vi "Get Product Info.vi"(8 "error in (no error)":errorcluster, 11 "Name":string) -> (0 "error out":errorcluster, 2 "success?":bool, 3 "Product Info":T1)   [LabVIEW 2020, in "SQLITE Inventory.lvlib"]
doc: "Gets the information of a single product query."
uses:
  SQLITE Inventory.lvlib
  Invetory Data Type.ctl
  <vilib>/drjdpowell/SQLite Library/SQL Connection/Open (path).vi
  <vilib>/drjdpowell/SQLite Library/SQL Connection/Open (string).vi
  <vilib>/AdvancedString/Path To Command Line String.vi
  <vilib>/drjdpowell/SQLite Library/SQL Connection/Execute SQL (Single Integer).vi
  <vilib>/drjdpowell/SQLite Library/SQL Connection/Connection.lvclass
  <vilib>/drjdpowell/SQLite Library/SQLite.lvlib
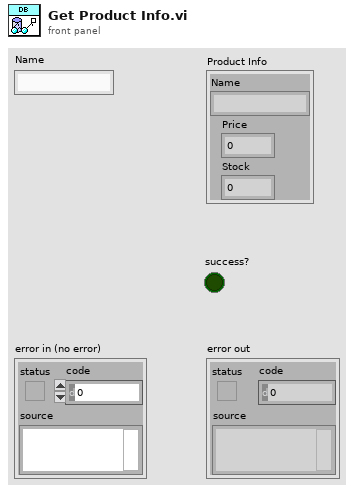
[diagram p1: front panel]
types:
  T1 = typedef "Invetory Data Type.ctl" = cluster{"Name":string, "Price":dbl, "Stock":dbl}
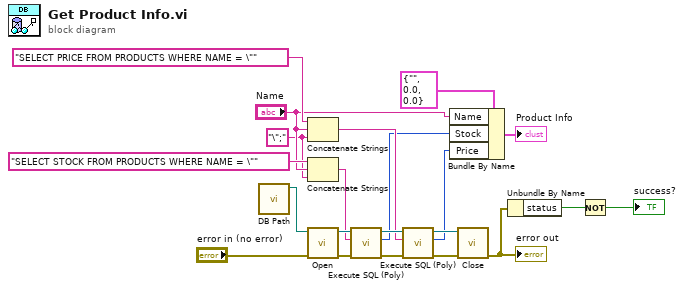
[diagram p0: block diagram]
diagram:
  w9 = "\";"
  n1 = call "DB Path.vi"() -> ("DB Path"=w21:path)  [unwired: 11 in]
  n2 = Concatenate Strings("SELECT PRICE FROM PRODUCTS WHERE NAME = \"" ("SQL"), "Name", w9) -> (w8:string)
  n3 = Concatenate Strings("SELECT STOCK FROM PRODUCTS WHERE NAME = \"" ("SQL"), "Name", w9) -> (w10:string)
  n4 = call-poly <vilib>:"Open.vi"("error in (no error)"="error in (no error)", "db file"=w21) -> ("error out"=w14:errorcluster, "SQLite Connection"=w13:refnum<class "Connection.lvclass">)  [unwired: 8 in]
  n5 = call-poly <vilib>:"Execute SQL (Poly).vi"("error in (no error)"=w14, "SQL"=w10, "SQLite Connection in"=w13) -> ("error out"=w12:errorcluster, "Result"=w6:i64, "SQLite Connection"=w11:refnum<class "Connection.lvclass">)  [unwired: 6 in]
  n6 = call-poly <vilib>:"Execute SQL (Poly).vi"("error in (no error)"=w12, "SQL"=w8, "SQLite Connection in"=w11) -> ("error out"=w19:errorcluster, "Result"=w5:i64, "SQLite Connection"=w20:refnum<class "Connection.lvclass">)  [unwired: 6 in]
  n7 = Bundle By Name(cluster=T1 {"Name"="", "Price"=0.0, "Stock"=0.0}, "Name"="Name", "Stock"=w6, "Price"=w5) -> (→"Product Info":T1)
  n8 = call-dynamic "Close.vi"("error in (no error)"=w19, "SQLite Connection in"=w20) -> ("error out"=w3:errorcluster)  [unwired: 9 in]
  "error out" <- w3
  n9 = Unbundle By Name(w3) -> ("status"=w2:bool)
  n10 = Not(x=w2) -> (.not. x?=→"success?":bool)
